vi "Provider_Interface.vi"() -> (3 "Interface Table":T1)   [LabVIEW 2020, in "Message Maker Provider.lvlib"]
uses:
  Message Maker Provider.lvlib
  <resource>/Framework/Providers/API/Provider_Interface.ctl
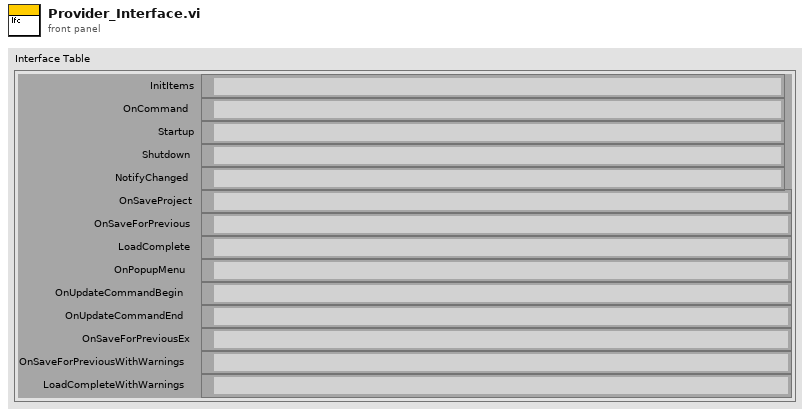
[diagram p1: front panel]
types:
  T1 = typedef "Provider_Interface.ctl" = cluster{"InitItems":path, "OnCommand":path, "Startup":path, "Shutdown":path, "NotifyChanged":path, "OnSaveProject":path, "OnSaveForPrevious":path, "LoadComplete":path, "OnPopupMenu":path, "OnUpdateCommandBegin":path, "OnUpdateCommandEnd":path, "OnSaveForPreviousEx":path, "OnSaveForPreviousWithWarnings":path, "LoadCompleteWithWarnings":path}
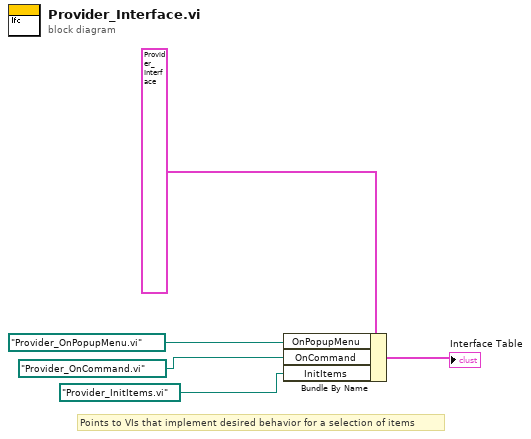
[diagram p0: block diagram]
diagram:
  # "Points to VIs that implement desired behavior for a selection of items"
  n1 = Bundle By Name(cluster=T1 {"InitItems"=path "", "OnCommand"=path "", "Startup"=path "", "Shutdown"=path "", "NotifyChanged"=path "", "OnSaveProject"=path "", "OnSaveForPrevious"=path "", "LoadComplete"=path "", "OnPopupMenu"=path "", "OnUpdateCommandBegin"=path "", "OnUpdateCommandEnd"=path "", "OnSaveForPreviousEx"=path "", "OnSaveForPreviousWithWarnings"=path "", "LoadCompleteWithWarnings"=path ""} ("InterfaceTable"), "OnPopupMenu"=path "Provider_OnPopupMenu.vi" ("string"), "OnCommand"=path "Provider_OnCommand.vi" ("string"), "InitItems"=path "Provider_InitItems.vi" ("string")) -> (→"Interface Table":T1)
